vi "Set configuration chain.vi"(8 "error in (no error)":errorcluster, 9 "class names":string[](array[string]), 10 "configuration":variant[](array[variant]), 11 "LineCCD in":refnum<class "LineCCD.lvclass">) -> (0 "error out":errorcluster, 3 "LineCCD out":refnum<class "LineCCD.lvclass">)   [LabVIEW 2012, in "LineCCD.lvclass"]
uses:
  LineCCD.lvclass
  <vilib>/Distrio/Murmex/Murmex/Murmex.lvclass
  LineCCD.lvclass/LineCCD.ctl
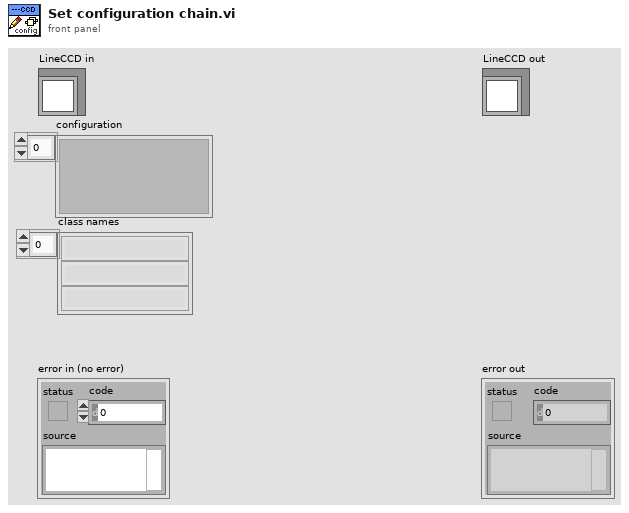
[diagram p1: front panel]
types:
  T1 = typedef "LineCCD.lvclass/configuration.ctl" = cluster{"Numeric":dbl}
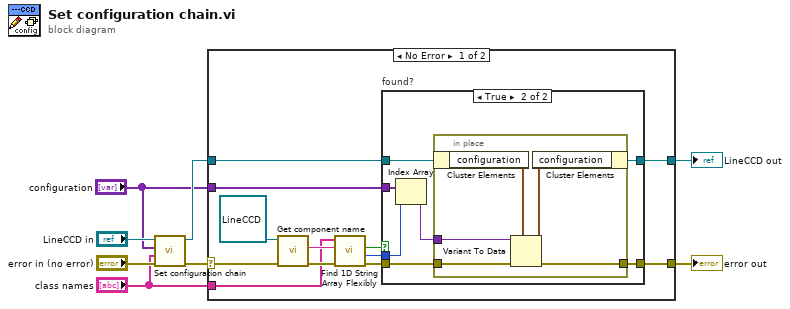
[diagram p0: block diagram]
diagram:
  n1 = call-parent "Set configuration chain.vi"("error in (no error)"="error in (no error)", "class names"="class names", "configuration"="configuration", "Murmex in"="LineCCD in") -> ("error out"=w6:errorcluster, "Murmex out"=w5:refnum<class "LineCCD.lvclass">)  [unwired: 6 in]
  n2 = case shown="No Error" w6 {
    selector: w6 -> [w15 w35]
    tunnel: w5 -> [w13 w36]
    tunnel: "configuration" -> [w12 _]
    tunnel: "class names" -> [w11 _]
    tunnel: [w10 w36] -> w2
    tunnel: [w9 w35] -> w1
    frame No Error {
      n3 = call <vilib>:"Get component name.vi"("error in (no error)"=w15, "Murmex in"=refnum<class "LineCCD.lvclass"> refnum ("LineCCD.lvclass")) -> ("error out"=w16:errorcluster, "component name"=w17:string)  [unwired: 7 in, 1 out]
      n4 = call <vilib>:"Find 1D String Array Flexibly.vi"("error in (no error)"=w16, "element"=w17, "array"=w11) -> ("error out"=w20:errorcluster, "index of element"=w19:i32, "found?"=w18:bool)  [unwired: 6 in]
      n5 = case "found?" shown="True" w18 {
        tunnel: w19 -> [_ w27]
        tunnel: w20 -> [w22 w26]
        tunnel: [w22 w25] -> w9
        tunnel: [w21 w23] -> w10
        tunnel: w13 -> [w21 w29]
        tunnel: w12 -> [_ w28]
        frame False {
        }
        frame True {
          n6 = Index Array(array=w28, index=w27) -> (element=w24:variant)
          n7 = in-place {
            in-place-border: w26 -> [w34]
            in-place-border: [w33] -> w25
            in-place-border: w24 -> [w30]
            n8 = in-place-cluster #1(w29) -> ("configuration"=w32:T1)
            n9 = Variant To Data(error in=w34, type=w32, Variant=w30) -> (data=w31:T1, error out=w33:errorcluster)
            n10 = in-place-cluster #1("configuration"=w31) -> (w23:refnum<class "LineCCD.lvclass">)
          }
        }
      }
    }
    frame Error {
    }
  }
  "error out" <- w1
  "LineCCD out" <- w2
